vi "ART-3029D-Read-DO.vi"(8 "error in (no error)":errorcluster) -> (0 "error out":errorcluster, 3 "Coils":bool[](array[boolean]))   [LabVIEW 2016, in "环境动力监测库.lvlib" / "浮标电源管理.lvlib"]
uses:
  <vilib>/Plasmionique/MB Master/MB_Master/MB_Master.lvclass
  <vilib>/Plasmionique/MB Master/MB Master.lvlib
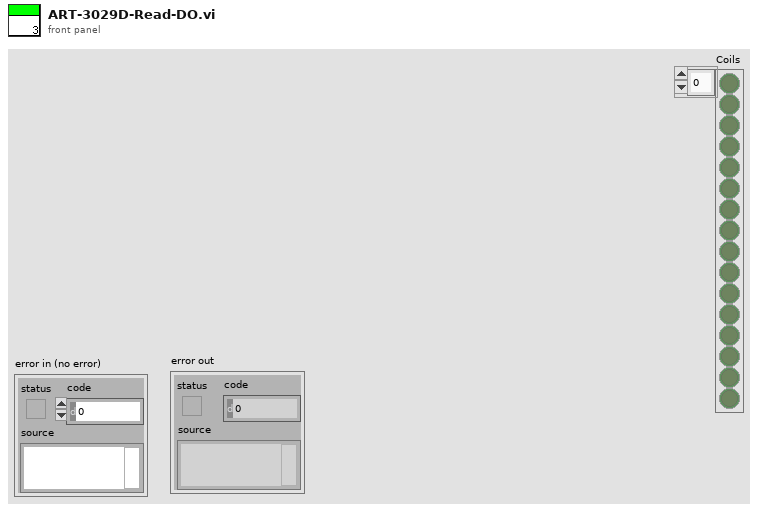
[diagram p1: front panel]
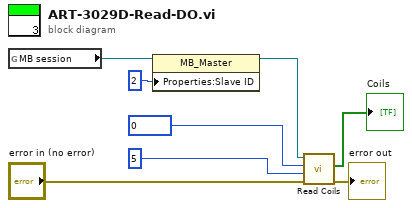
[diagram p0: block diagram]
diagram:
  n1 = global read "通讯全局变量.vi" "MB session"() -> (w5:refnum<class "MB_Master.lvclass">)
  n2 = property class="MB_Master"(reference=w5, "Properties:Slave ID"=u8 2 ("Slave ID")) -> (reference out=w4:refnum<class "MB_Master.lvclass">)  [unwired: 1 in, 1 out]
  n3 = call <vilib>:"Read Coils.vi"("error in (no error)"="error in (no error)", "quantity"=u16 5, "starting address"=u16 0, "MB session in"=w4) -> ("error out"=→"error out":errorcluster, "Coils"=→"Coils":bool[])  [unwired: 5 in, 1 out]
